vi "PID Parameters.vi"(8 "error in (no error)":errorcluster, 11 "Node Ptr":T1 format="%.0x") -> (0 "error out":errorcluster)   [LabVIEW 2019, in "Control Addon System Explorer.lvlib"]
uses:
  Control Addon System Explorer.lvlib
  <vilib>/NI VeriStand/Custom Device API/Custom Device API.lvlib
  Addon Shared/Constants.vi
  Addon Shared/Control Addon Shared.lvlib
  Types/Action.ctl
  <vilib>/NI VeriStand/Custom Device API/Custom Device Item Ref.ctl
  NationalInstruments.VeriStand.SystemStorageUI
panel:
  in  "Export":bool
  in  "Import":bool
  in  "Reset":bool
  in  "Apply":bool
  in  "Header 3":cluster{"Section Name":string}={"Section Name"="PID Settings"}
  in  "Enable Live Updates":bool
  in  "PID Settings":i32(listbox)
  in  "Gain Schedule Channel":refnum<k24>(container) caption="Gain Schedule Signal"
  in  "Header 2":cluster{"Section Name":string}={"Section Name"="Gain Schedule Settings"}
  in  "Enable Gain Scheduling":bool
  in  "SHDocVw.IWebBrowser":refnum<k7>(container)
  in  "Header":cluster{"Section Name":string}={"Section Name"="Custom Device Item Settings"}
  in  "Description":string
  out "Name":string
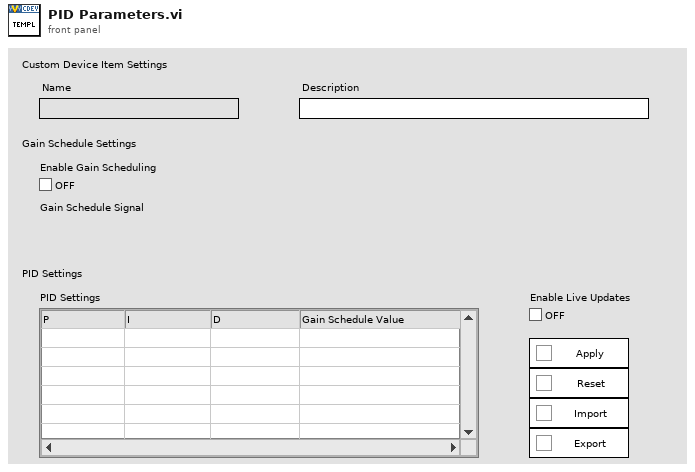
[diagram p1: front panel]
types:
  T1 = typedef "Custom Device API.lvlib/Custom Device Item Ref.ctl" = u64
  T2 = typedef "Control Addon System Explorer.lvlib/Action.ctl" = enum16{"Get", "Set"}
  T3 = typedef "Control Addon Shared.lvlib/PID Parameters.ctl" = cluster{"Enable Live Updates":bool, "Enable Gain Scheduling":bool, "PID Parameters":dbl[][]}
  T4 = typedef "Control Addon System Explorer.lvlib/PID Parameters Channel Browser Refs.ctl" = cluster{"GainSchedule":refnum<user-event>}
  T5 = typedef "Custom Device API.lvlib/Custom Device Item Info.ctl" = cluster{"Name":string, "Is Channel":bool, "GUID":string, "Is Waveform":bool}
  T6 = typedef "Custom Device API.lvlib/Custom Device Commands.ctl" = enum16{"Default", "Item renamed", "Shutdown", "Dynamic button pressed"}
  T7 = typedef "LVPoint32TypeDef.ctl" = cluster{"Horizontal":i32, "Vertical":i32}
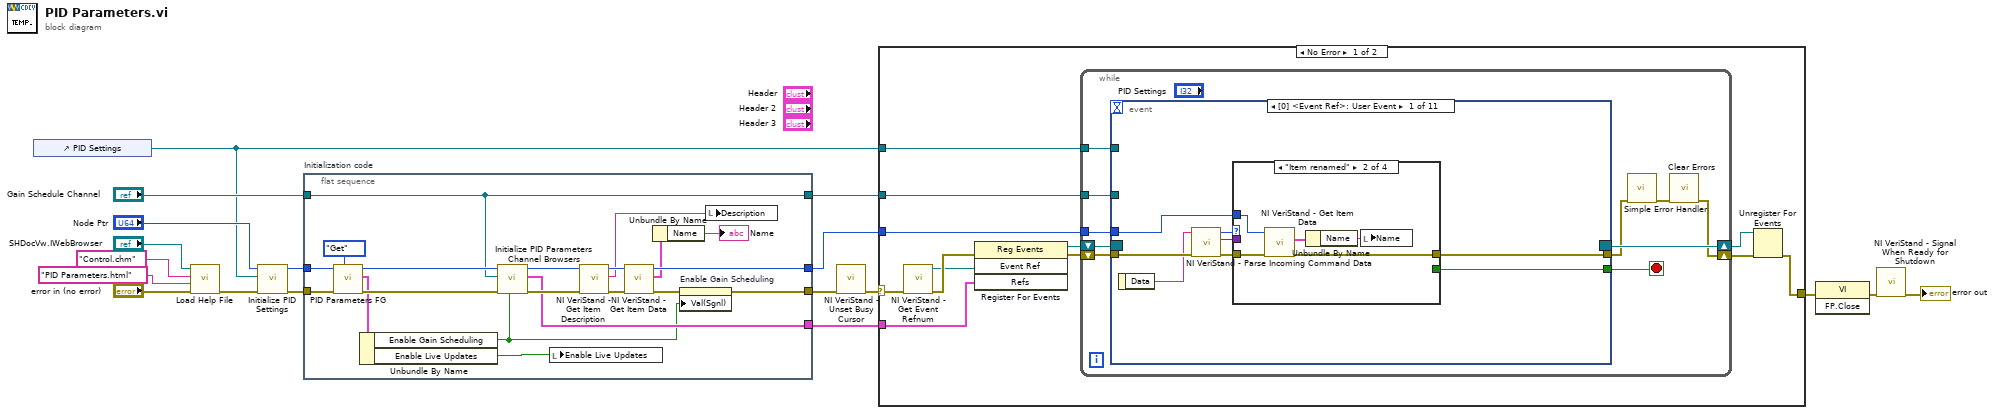
[diagram p0: block diagram]
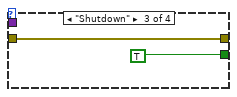
[diagram p3: hidden frame]
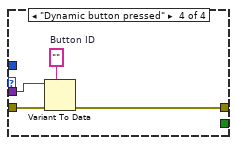
[diagram p4: hidden frame]
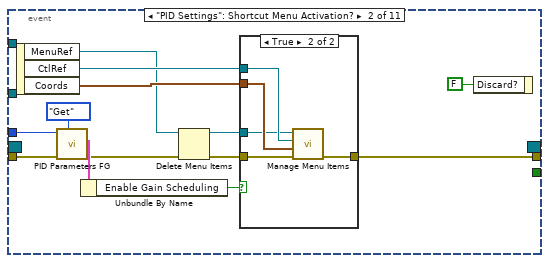
[diagram p5: hidden frame]
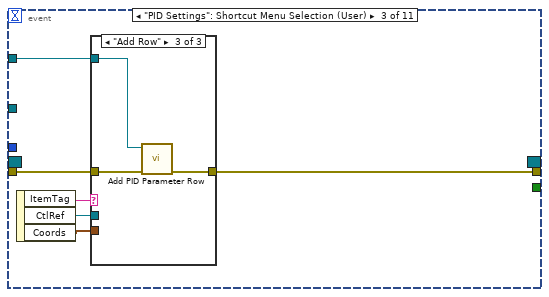
[diagram p7: hidden frame]
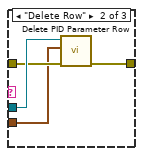
[diagram p9: hidden frame]
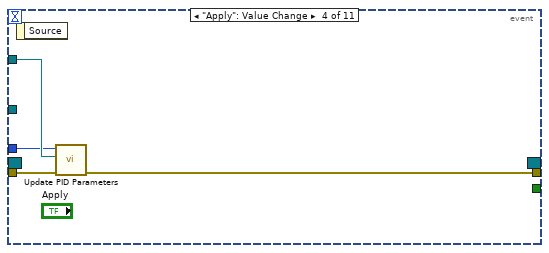
[diagram p10: hidden frame]
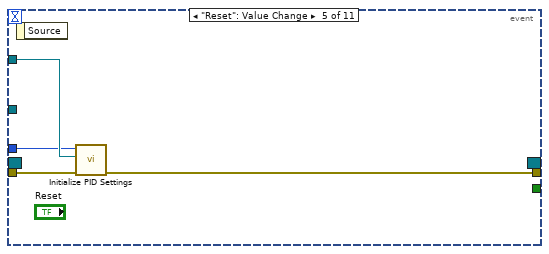
[diagram p11: hidden frame]
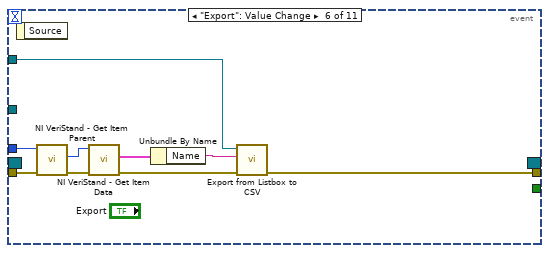
[diagram p12: hidden frame]
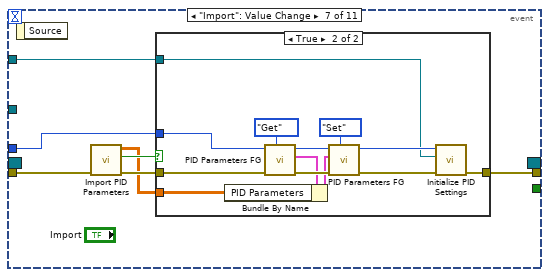
[diagram p13: hidden frame]
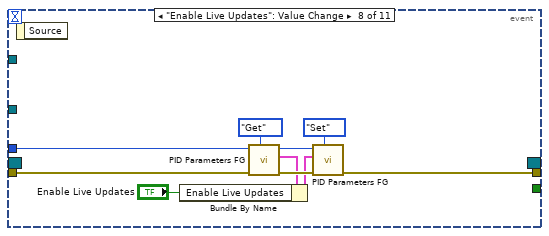
[diagram p15: hidden frame]
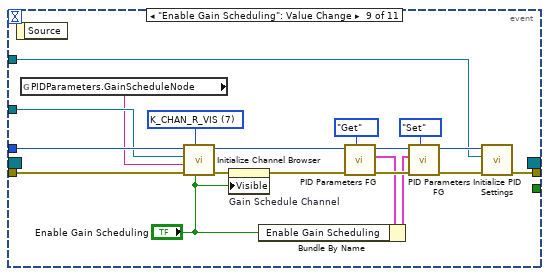
[diagram p16: hidden frame]
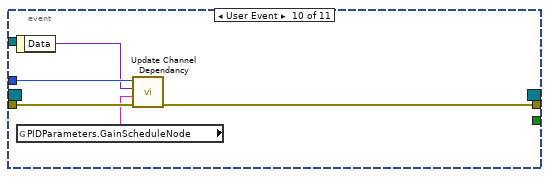
[diagram p17: hidden frame]
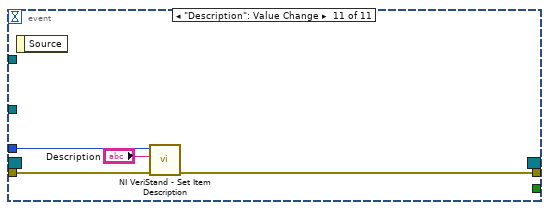
[diagram p18: hidden frame]
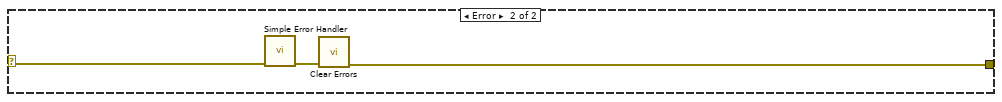
[diagram p19: hidden frame]
diagram:
  n1 = control-ref of="PID Settings"() -> (w2:refnum<vi>)
  n2 = call "Load Help File.vi"("error in (no error)"="error in (no error)", "HTML File"="PID Parameters.html", "Main CHM File"="Control.chm", "SHDocVw.IWebBrowser2"="SHDocVw.IWebBrowser") -> ("error out"=w6:errorcluster)  [unwired: 7 in]
  n3 = call "Initialize PID Settings.vi"("error in (no error)"=w6, "PID Settings"=w2, "Item Ref in"="Node Ptr") -> ("error out"=w5:errorcluster, "Item Ref out"=w3:T1)  [unwired: 7 in]
  n4 = flat-sequence "Initialization code" {
    tunnel: w5 -> [w32]
    tunnel: w3 -> [w30]
    tunnel: [w23] -> w15
    tunnel: [w38] -> w13
    tunnel: "Gain Schedule Channel" -> [w19]
    tunnel: [w25] -> w7
    tunnel: [w19] -> w1
    frame #0 {
      n5 = call "PID Parameters FG.vi"("Action"=Action."Get", "error in (no error)"=w32, "Node Ptr"=w30) -> ("error out"=w31:errorcluster, "Parameters"=w28:T3, "Item Ref out"=w22:T1)  [unwired: 6 in]
      n6 = Unbundle By Name(w28) -> ("Enable Gain Scheduling"=w21:bool, "Enable Live Updates"=w27:bool)
      n7 = call "Initialize PID Parameters Channel Browsers.vi"("Enable Gain Scheduling"=w21, "error in (no error)"=w31, "Channel Browser"=w19, "Item Ref in"=w22) -> ("error out"=w26:errorcluster, "Refs"=w25:T4, "Item Ref out"=w20:T1)  [unwired: 5 in]
      n8 = local write "Enable Live Updates"(w27) -> ()
      n9 = call <vilib>:"NI VeriStand - Get Item Description.vi"("error in (no error)"=w26, "Item Ref in"=w20) -> ("error out"=w35:errorcluster, "Description"=w36:string, "Item Ref out"=w37:T1)  [unwired: 7 out]
      n10 = call <vilib>:"NI VeriStand - Get Item Data.vi"("error in (no error)"=w35, "Item Ref in"=w37) -> ("error out"=w24:errorcluster, "Item Info"=w34:T5, "Item Ref out"=w38:T1)  [unwired: 7 out]
      n11 = Unbundle By Name(w34) -> ("Name"=→"Name":string)
      n12 = property on="Enable Gain Scheduling" class="Bool (strict)"(error in=w24, "Val(Sgnl)"=w21) -> (error out=w23:errorcluster)  [unwired: 1 in, 1 out]
      n13 = local write "Description"(w36) -> ()
    }
  }
  n14 = call <vilib>:"NI VeriStand - Unset Busy Cursor.vi"("error in (no error)"=w15) -> ("error out"=w14:errorcluster)  [unwired: 10 out]
  n15 = case shown="No Error" w14 {
    selector: w14 -> [w42 w192]
    tunnel: [w47 w190] -> w18
    tunnel: w13 -> [w43 _]
    tunnel: w7 -> [w41 _]
    tunnel: w2 -> [w40 _]
    tunnel: w1 -> [w39 _]
    frame No Error {
      n16 = call <vilib>:"NI VeriStand - Get Event Refnum.vi"("error in (no error)"=w42) -> ("error out"=w50:errorcluster, "Event Ref"=w46:refnum<user-event>)  [unwired: 9 out]
      n17 = register-events(error in=w50, w46, w41) -> (reference out=w44:refnum<event-registration>, error out=w45:errorcluster)  [unwired: 1 in]
      n18 = while {
        tunnel: w43 -> [w56]
        shift-right: [w53] -> w48
        shift-left: w45 -> [w59]
        shift-right: [w60] -> w49
        shift-left: w44 -> [w58]
        tunnel: w40 -> [w52]
        tunnel: w39 -> [w51]
        stop <- w57 stop-if-true
        n19 = event shown="[0] <Event Ref>: User Event" {
          selector: w58 -> [_ _ _ _ _ _ _ _ _ _ _]
          dyn-events: [_ _ _ _ _ _ _ _ _ _ _] -> w60
          timeout: _ -> [_ _ _ _ _ _ _ _ _ _ _]
          tunnel: w59 -> [w68 w88 w105 w117 w121 w128 w137 w160 w172 w185 w188]
          tunnel: [w64 _ _ _ _ _ _ _ _ _ _] -> w57
          tunnel: [w63 w90 w102 w116 w118 w129 w135 w152 w164 w181 w187] -> w55
          tunnel: w56 -> [w62 w87 _ w114 w119 w130 w132 w159 w170 w184 w189]
          tunnel: w52 -> [_ _ w103 w115 w120 w122 w131 _ w162 _ _]
          tunnel: w51 -> [_ _ _ _ _ _ _ _ w167 _ _]
          event User Event {
            n20 = event-data() -> ("Data"=w67:string)  [unwired: 1 out]
            n21 = call <vilib>:"NI VeriStand - Parse Incoming Command Data.vi"("error in (no error)"=w68, "Incoming data"=w67) -> ("error out"=w66:errorcluster, "Outgoing data"=w61:variant, "Action"=w65:T6)  [unwired: 7 out]
            n22 = case shown="\"Item renamed\"" w65 {
              tunnel: w66 -> [w69 w74 w75 w80]
              tunnel: [_ _ TRUE _] -> w64
              tunnel: [w69 w71 w75 w77] -> w63
              tunnel: w62 -> [_ w73 _ _]
              tunnel: w61 -> [_ _ _ w79]
              frame "Default", Default {
              }
              frame "Item renamed" {
                n23 = call <vilib>:"NI VeriStand - Get Item Data.vi"("error in (no error)"=w74, "Item Ref in"=w73) -> ("error out"=w71:errorcluster, "Item Info"=w72:T5)  [unwired: 8 out]
                n24 = Unbundle By Name(w72) -> ("Name"=w70:string)
                n25 = local write "Name"(w70) -> ()
              }
              frame "Shutdown" {
              }
              frame "Dynamic button pressed" {
                w78 = ""  # Button ID
                n26 = Variant To Data(error in=w80, type=w78, Variant=w79) -> (error out=w77:errorcluster)  [unwired: 1 out]
              }
            }
          }
          event "PID Settings": Shortcut Menu Activation? {
            n27 = event-data() -> ("MenuRef"=w82:refnum<k9>, "CtlRef"=w93:refnum<vi>, "Coords"=w92:T7)  [unwired: 1 out]
            n28 = call "PID Parameters FG.vi"("Action"=Action."Get", "error in (no error)"=w88, "Node Ptr"=w87) -> ("error out"=w84:errorcluster, "Parameters"=w86:T3)  [unwired: 6 in, 1 out]
            n29 = Unbundle By Name(w86) -> ("Enable Gain Scheduling"=w85:bool)
            n30 = Delete Menu Items(6:w84, 9:w82) -> (0:w83:errorcluster, 3:w81:refnum<k9>)  [unwired: 2 in]
            n31 = case shown="True" w85 {
              tunnel: w93 -> [_ w99]
              tunnel: w92 -> [_ w98]
              tunnel: w81 -> [_ w97]
              tunnel: [w94 w96] -> w90
              tunnel: w83 -> [w94 w95]
              frame False {
              }
              frame True {
                n32 = call "Manage Menu Items.vi"("error in (no error)"=w95, "Coords"=w98, "CtlRef"=w99, "Menu in"=w97) -> ("error out"=w96:errorcluster)  [unwired: 7 in]
              }
            }
            n33 = event-data("Discard?"=FALSE) -> ()  [unwired: 1 in, 1 out]
          }
          event "PID Settings": Shortcut Menu Selection (User) {
            n34 = event-data() -> ("ItemTag"=w104:string, "CtlRef"=w101:refnum<vi>, "Coords"=w100:T7)  [unwired: 1 out]
            n35 = case shown="\"Add Row\"" w104 {
              tunnel: w105 -> [w106 w109 w113]
              tunnel: w103 -> [_ _ w112]
              tunnel: [w106 w107 w111] -> w102
              tunnel: w101 -> [_ w110 _]
              tunnel: w100 -> [_ w108 _]
              frame Default {
              }
              frame "Delete Row" {
                n36 = call "Delete PID Parameter Row.vi"("error in (no error)"=w109, "Coords"=w108, "MulticolumnListbox in"=w110) -> ("error out"=w107:errorcluster)  [unwired: 8 in]
              }
              frame "Add Row" {
                n37 = call "Add PID Parameter Row.vi"("error in (no error)"=w113, "MulticolumnListbox in"=w112) -> ("error out"=w111:errorcluster)  [unwired: 9 in]
              }
            }
          }
          event "Apply": Value Change {
            n38 = event-data() -> ()  [unwired: 2 out]
            n39 = call "Update PID Parameters.vi"("error in (no error)"=w117, "PID Settings"=w115, "Item Ref in"=w114) -> ("error out"=w116:errorcluster)  [unwired: 7 in, 1 out]
          }
          event "Reset": Value Change {
            n40 = event-data() -> ()  [unwired: 2 out]
            n41 = call "Initialize PID Settings.vi"("error in (no error)"=w121, "PID Settings"=w120, "Item Ref in"=w119) -> ("error out"=w118:errorcluster)  [unwired: 7 in, 1 out]
          }
          event "Export": Value Change {
            n42 = event-data() -> ()  [unwired: 2 out]
            n43 = call <vilib>:"NI VeriStand - Get Item Parent.vi"("error in (no error)"=w128, "Item Ref in"=w130) -> ("error out"=w126:errorcluster, "Parent Ref"=w127:T1)  [unwired: 6 in, 2 out]
            n44 = call <vilib>:"NI VeriStand - Get Item Data.vi"("error in (no error)"=w126, "Item Ref in"=w127) -> ("error out"=w123:errorcluster, "Item Info"=w125:T5)  [unwired: 8 out]
            n45 = Unbundle By Name(w125) -> ("Name"=w124:string)
            n46 = call "Export from Listbox to CSV.vi"("error in (no error)"=w123, "Name"=w124, "MulticolumnListbox in"=w122) -> ("error out"=w129:errorcluster)  [unwired: 8 in]
          }
          event "Import": Value Change {
            n47 = event-data() -> ()  [unwired: 2 out]
            n48 = call "Import PID Parameters.vi"("error in"=w137) -> ("error out"=w134:errorcluster, "Apply?"=w136:bool, "Parameters"=w133:dbl[][])  [unwired: 8 in]
            n49 = case shown="True" w136 {
              tunnel: [w138 w140] -> w135
              tunnel: w134 -> [w138 w144]
              tunnel: w133 -> [_ w145]
              tunnel: w132 -> [_ w143]
              tunnel: w131 -> [_ w139]
              frame False {
              }
              frame True {
                n50 = call "PID Parameters FG.vi"("Action"=Action."Get", "error in (no error)"=w144, "Node Ptr"=w143) -> ("error out"=w149:errorcluster, "Parameters"=w147:T3, "Item Ref out"=w148:T1)  [unwired: 6 in]
                n51 = Bundle By Name(cluster=w147, "PID Parameters"=w145) -> (w146:T3)
                n52 = call "PID Parameters FG.vi"("Action"=Action."Set", "error in (no error)"=w149, "Parameters"=w146, "Node Ptr"=w148) -> ("error out"=w141:errorcluster, "Item Ref out"=w142:T1)  [unwired: 5 in, 1 out]
                n53 = call "Initialize PID Settings.vi"("error in (no error)"=w141, "PID Settings"=w139, "Item Ref in"=w142) -> ("error out"=w140:errorcluster)  [unwired: 7 in, 1 out]
              }
            }
          }
          event "Enable Live Updates": Value Change {
            n54 = event-data() -> ()  [unwired: 2 out]
            n55 = call "PID Parameters FG.vi"("Action"=Action."Get", "error in (no error)"=w160, "Node Ptr"=w159) -> ("error out"=w157:errorcluster, "Parameters"=w155:T3, "Item Ref out"=w156:T1)  [unwired: 6 in]
            n56 = Bundle By Name(cluster=w155, "Enable Live Updates"="Enable Live Updates") -> (w154:T3)
            n57 = call "PID Parameters FG.vi"("Action"=Action."Set", "error in (no error)"=w157, "Parameters"=w154, "Node Ptr"=w156) -> ("error out"=w152:errorcluster)  [unwired: 5 in, 2 out]
          }
          event "Enable Gain Scheduling": Value Change {
            w173 = u8 7 items=["K_CHAN_R", "K_CHAN_W", "K_CHAN_RW", "K_CHAN_VOLT", "K_CHAN_FAULT", "K_ALL", "K_CUSTOM", "K_CHAN_R_VIS", "K_CHAN_W_VIS", "K_CHAN_RW_VIS", "K_CHAN_VOLT_VIS", "K_CHAN_FAULT_VIS"] ("DisplayFilter")
            n58 = event-data() -> ()  [unwired: 2 out]
            n59 = global read "Constants.vi" "PIDParameters.GainScheduleNode"() -> (w166:string)
            n60 = call "Initialize Channel Browser.vi"("Use Channel?"="Enable Gain Scheduling", "DisplayFilter"=w173, "error in (no error)"=w172, "NodeName"=w166, "Browser Ref"=w167, "Item Ref in"=w170) -> ("error out"=w171:errorcluster, "Item Ref out"=w169:T1)  [unwired: 3 in, 1 out]
            n61 = property on="Gain Schedule Channel" class="AXCont"(error in=w171, "Visible"="Enable Gain Scheduling") -> (error out=w174:errorcluster)  [unwired: 1 in, 1 out]
            n62 = call "PID Parameters FG.vi"("Action"=Action."Get", "error in (no error)"=w174, "Node Ptr"=w169) -> ("error out"=w178:errorcluster, "Parameters"=w176:T3, "Item Ref out"=w177:T1)  [unwired: 6 in]
            n63 = Bundle By Name(cluster=w176, "Enable Gain Scheduling"="Enable Gain Scheduling") -> (w175:T3)
            n64 = call "PID Parameters FG.vi"("Action"=Action."Set", "error in (no error)"=w178, "Parameters"=w175, "Node Ptr"=w177) -> ("error out"=w165:errorcluster, "Item Ref out"=w163:T1)  [unwired: 5 in, 1 out]
            n65 = call "Initialize PID Settings.vi"("error in (no error)"=w165, "PID Settings"=w162, "Item Ref in"=w163) -> ("error out"=w164:errorcluster)  [unwired: 7 in, 1 out]
          }
          event User Event {
            n66 = event-data() -> ("Data"=w183:variant)  [unwired: 1 out]
            n67 = global read "Constants.vi" "PIDParameters.GainScheduleNode"() -> (w182:string)
            n68 = call "Update Channel Dependancy.vi"("error in (no error)"=w185, "NodeName"=w182, "Data"=w183, "Item Ref in"=w184) -> ("error out"=w181:errorcluster)  [unwired: 6 in, 1 out]
          }
          event "Description": Value Change {
            n69 = event-data() -> ()  [unwired: 2 out]
            n70 = call <vilib>:"NI VeriStand - Set Item Description.vi"("error in (no error)"=w188, "Description"="Description", "Item Ref in"=w189) -> ("error out"=w187:errorcluster)  [unwired: 8 out]
          }
        }
        n71 = call <vilib>:"Simple Error Handler.vi"("error in (no error)"=w55) -> ("error out"=w54:errorcluster)  [unwired: 1 in, 7 out]
        n72 = call <vilib>:"Clear Errors.vi"("error in (no error)"=w54) -> ("error out"=w53:errorcluster)  [unwired: 1 in, 5 out]
      }
      n73 = Unregister For Events(event registration refnum=w49, error in=w48) -> (error out=w47:errorcluster)
    }
    frame Error {
      n74 = call <vilib>:"Simple Error Handler.vi"("error in (no error)"=w192) -> ("error out"=w191:errorcluster)  [unwired: 1 in, 7 out]
      n75 = call <vilib>:"Clear Errors.vi"("error in (no error)"=w191) -> ("error out"=w190:errorcluster)  [unwired: 1 in, 5 out]
    }
  }
  n76 = invoke class="VI" method="FP.Close"(error in=w18) -> (error out=w17:errorcluster)  [unwired: 2 in, 2 out]
  n77 = call <vilib>:"NI VeriStand - Signal When Ready for Shutdown.vi"("error in (no error)"=w17) -> ("error out"=→"error out":errorcluster)  [unwired: 10 out]
